vi "test Get-Set-Get Parameter Definitions.vi"(8 "error in":errorcluster, 11 "TestCase in":refnum<class "Scripting.lvclass">) -> (0 "error out":errorcluster, 3 "TestCase out":refnum<class "Scripting.lvclass">)   [LabVIEW 2023, in "Scripting.lvclass"]
uses:
  Scripting.lvclass
  <vilib>/addons/_JKI Toolkits/VI Tester/TestCase.llb/TestCase.lvclass
  Scripting/Ballard MIL-STD-1553 Scripting.lvlib
  Shared/Address.ctl
  Shared/Message Type.ctl
  Shared/Terminal Endpoint.ctl
  Shared/Parameter Definition.ctl
  Shared/Message Definition.ctl
  Shared/1553 Channel.ctl
  <vilib>/NI VeriStand/Custom Device API/Custom Device API.lvlib
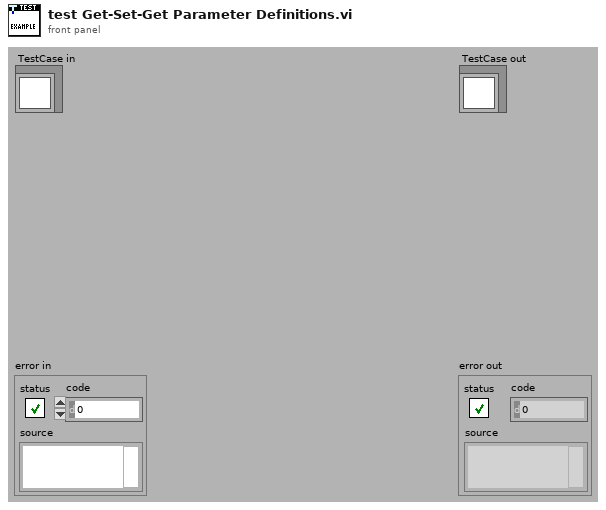
[diagram p1: front panel]
types:
  T1 = typedef "1553 Channel.ctl" = cluster{"HW channel":u16, "bus controller":cluster{"simulated?":bool, "name":string}, "terminal addresses":T2[], "terminal names":string[], "acyclic frame names":string[], "messages":T3[]}
  T2 = typedef "Address.ctl" = u16
  T3 = typedef "Message Definition.ctl" = cluster{"name":string, "message type":T4, "endpoint Tx":T5, "endpoint Rx":T5, "create timestamp channel":bool, "mode code":u16, "number of words":u16, "parameters":cluster{"name":string, "default value":dbl, "unit":string, "parameter definition":T6}[]}
  T4 = typedef "Message Type.ctl" = string
  T5 = typedef "Terminal Endpoint.ctl" = cluster{"terminal address":T2, "subaddress":T2}
  T6 = typedef "Parameter Definition.ctl" = cluster{"start index":i32, "size (bits)":i32, "encoding":enum16{"BNR", "BCD", "Discrete"}, "signed":bool, "multiplier":dbl, "offset":dbl}
  T7 = typedef "Custom Device API.lvlib/Custom Device Item Ref.ctl" = u64
  T8 = cluster{"name":string, "default value":dbl, "unit":string, "parameter definition":T6}[]
  T9 = typedef "Custom Device API.lvlib/Custom Device Channel.ctl" = cluster{"Type":T10, "Units":string, "Default Value":dbl, "Faultable":bool, "Scalable":bool}
  T10 = typedef "Custom Device API.lvlib/Custom Device Channel Type.ctl" = enum16{"Input", "Output"}
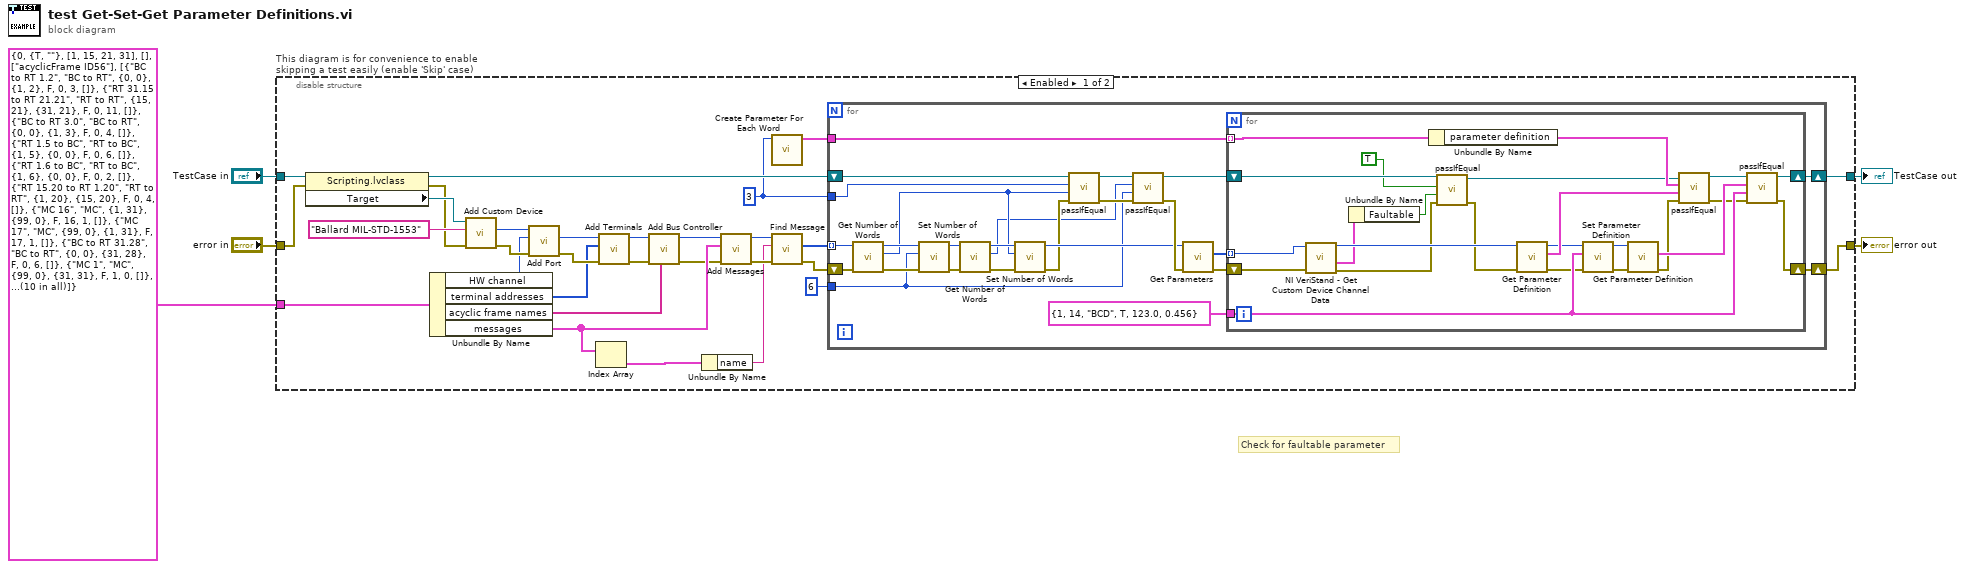
[diagram p0: block diagram]
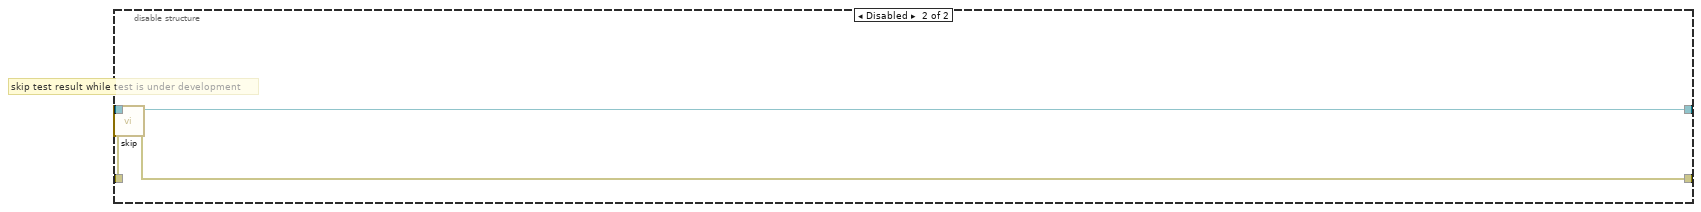
[diagram p2: hidden frame]
diagram:
  # "Check for faultable parameter"
  n1 = disable-structure "This diagram is for convenience to enable skipping a test easily (enable 'Skip' case)" shown="Enabled" {
    disable-tunnel: "TestCase in" -> [w34 w88]
    disable-tunnel: [w15 w86] -> w2
    disable-tunnel: [w14 w87] -> w4
    disable-tunnel: "error in" -> [w19 w85]
    disable-tunnel: T1 {"HW channel"=0, "bus controller"={"simulated?"=TRUE, "name"=""}, "terminal addresses"=[1, 15, 21, 31], "terminal names"=[], "acyclic frame names"=["acyclicFrame ID56"], "messages"=[{"name"="BC to RT 1.2", "message type"="BC to RT", "endpoint Tx"={"terminal address"=0, "subaddress"=0}, "endpoint Rx"={"terminal address"=1, "subaddress"=2}, "create timestamp channel"=FALSE, "mode code"=0, "number of words"=3, "parameters"=[]}, {"name"="RT 31.15 to RT 21.21", "message type"="RT to RT", "endpoint Tx"={"terminal address"=15, "subaddress"=21}, "endpoint Rx"={"terminal address"=31, "subaddress"=21}, "create timestamp channel"=FALSE, "mode code"=0, "number of words"=11, "parameters"=[]}, {"name"="BC to RT 3.0", "message type"="BC to RT", "endpoint Tx"={"terminal address"=0, "subaddress"=0}, "endpoint Rx"={"terminal address"=1, "subaddress"=3}, "create timestamp channel"=FALSE, "mode code"=0, "number of words"=4, "parameters"=[]}, {"name"="RT 1.5 to BC", "message type"="RT to BC", "endpoint Tx"={"terminal address"=1, "subaddress"=5}, "endpoint Rx"={"terminal address"=0, "subaddress"=0}, "create timestamp channel"=FALSE, "mode code"=0, "number of words"=6, "parameters"=[]}, {"name"="RT 1.6 to BC", "message type"="RT to BC", "endpoint Tx"={"terminal address"=1, "subaddress"=6}, "endpoint Rx"={"terminal address"=0, "subaddress"=0}, "create timestamp channel"=FALSE, "mode code"=0, "number of words"=2, "parameters"=[]}, {"name"="RT 15.20 to RT 1.20", "message type"="RT to RT", "endpoint Tx"={"terminal address"=1, "subaddress"=20}, "endpoint Rx"={"terminal address"=15, "subaddress"=20}, "create timestamp channel"=FALSE, "mode code"=0, "number of words"=4, "parameters"=[]}, {"name"="MC 16", "message type"="MC", "endpoint Tx"={"terminal address"=1, "subaddress"=31}, "endpoint Rx"={"terminal address"=99, "subaddress"=0}, "create timestamp channel"=FALSE, "mode code"=16, "number of words"=1, "parameters"=[]}, {"name"="MC 17", "message type"="MC", "endpoint Tx"={"terminal address"=99, "subaddress"=0}, "endpoint Rx"={"terminal address"=1, "subaddress"=31}, "create timestamp channel"=FALSE, "mode code"=17, "number of words"=1, "parameters"=[]}, {"name"="BC to RT 31.28", "message type"="BC to RT", "endpoint Tx"={"terminal address"=0, "subaddress"=0}, "endpoint Rx"={"terminal address"=31, "subaddress"=28}, "create timestamp channel"=FALSE, "mode code"=0, "number of words"=6, "parameters"=[]}, {"name"="MC 1", "message type"="MC", "endpoint Tx"={"terminal address"=99, "subaddress"=0}, "endpoint Rx"={"terminal address"=31, "subaddress"=31}, "create timestamp channel"=FALSE, "mode code"=1, "number of words"=0, "parameters"=[]}]} ("1553 channel") -> [w11 _]
    frame Enabled {
      w17 = u16 3 ("number of words")
      n2 = property class="Scripting.lvclass"(reference=w34, error in=w19) -> (reference out=w20:refnum<class "Scripting.lvclass">, error out=w18:errorcluster, "Target"=w33:refnum<k24>)
      n3 = Unbundle By Name(w11) -> ("HW channel"=w29:u16, "terminal addresses"=w26:T2[], "acyclic frame names"=w6:string[], "messages"=w12:T3[])
      n4 = call "Add Custom Device.vi"("error in"=w18, "name"="Ballard MIL-STD-1553", "target in"=w33) -> ("error out"=w32:errorcluster, "Ballard MIL-STD 1553 custom device"=w31:T7)  [unwired: 6 in, 1 out]
      n5 = call "Add Port.vi"("error in"=w32, "port number"=w29, "Ballard MIL-STD 1553 custom device in"=w31) -> ("error out"=w27:errorcluster, "port"=w28:T7)  [unwired: 6 in, 1 out]
      n6 = Index Array(array=w12) -> (element=w23:T3)  [unwired: 1 in]
      n7 = call "Add Terminals.vi"("error in"=w27, "terminal addresses"=w26, "port in"=w28) -> ("error out"=w10:errorcluster, "port out"=w9:T7)  [unwired: 7 in]
      n8 = call "Add Bus Controller.vi"("acyclic frame names"=w6, "error in"=w10, "port in"=w9) -> ("error out"=w7:errorcluster, "port out"=w8:T7)  [unwired: 6 in, 1 out]
      n9 = Unbundle By Name(w23) -> ("name"=w24:string)
      n10 = call "Add Messages.vi"("error in"=w7, "messages"=w12, "port in"=w8) -> ("error out"=w25:errorcluster, "port out"=w30:T7)  [unwired: 7 in]
      n11 = call "Create Parameter For Each Word.vi"("number of words"=w17) -> ("parameters"=w16:T8)  [unwired: 9 in, 1 out]
      n12 = call "Find Message.vi"("error in"=w25, "message name"=w24, "port in"=w30) -> ("error out"=w21:errorcluster, "message refs"=w22:T7[])  [unwired: 5 in, 2 out]
      n13 = for {
        tunnel: w22 -> [w60] mode=indexing
        shift-right: [w45] -> w14
        shift-left: w21 -> [w59]
        shift-right: [w46] -> w15
        shift-left: w20 -> [w52]
        tunnel: w17 -> [w40]
        tunnel: w16 -> [w48]
        tunnel: u16 6 ("number of words") -> [w37]
        n14 = call "Get Number of Words.vi"("error in"=w59, "message in"=w60) -> ("error out"=w57:errorcluster, "number of words"=w38:u16, "message out"=w58:T7)  [unwired: 7 in]
        n15 = call "Set Number of Words.vi"("error in"=w57, "number of words"=w37, "message in"=w58) -> ("error out"=w56:errorcluster, "message out"=w55:T7)  [unwired: 7 in]
        n16 = call "Get Number of Words.vi"("error in"=w56, "message in"=w55) -> ("error out"=w42:errorcluster, "number of words"=w36:u16, "message out"=w44:T7)  [unwired: 7 in]
        n17 = call "Set Number of Words.vi"("error in"=w42, "number of words"=w38, "message in"=w44) -> ("error out"=w41:errorcluster, "message out"=w43:T7)  [unwired: 7 in]
        n18 = call-dynamic "passIfEqual.vi"("error in (no error)"=w41, "y"=w38, "x"=w40, "TestCase in"=w52) -> ("error out"=w54:errorcluster, "TestCase out"=w53:refnum<class "Scripting.lvclass">)  [unwired: 6 in]
        n19 = call-dynamic "passIfEqual.vi"("error in (no error)"=w54, "y"=w37, "x"=w36, "TestCase in"=w53) -> ("error out"=w51:errorcluster, "TestCase out"=w47:refnum<class "Scripting.lvclass">)  [unwired: 6 in]
        n20 = call "Get Parameters.vi"("error in"=w51, "message in"=w43) -> ("error out"=w50:errorcluster, "parameters"=w49:T7[])  [unwired: 7 in, 1 out]
        n21 = for {
          shift-right: [w76] -> w45
          shift-left: w50 -> [w70]
          tunnel: w49 -> [w68] mode=indexing
          tunnel: w48 -> [w75] mode=indexing
          shift-right: [w77] -> w46
          shift-left: w47 -> [w66]
          tunnel: T6 {"start index"=1, "size (bits)"=14, "encoding"=enum."BCD", "signed"=TRUE, "multiplier"=123.0, "offset"=0.456} ("parameter definition") -> [w79]
          n22 = call <vilib>:"NI VeriStand - Get Custom Device Channel Data.vi"("error in (no error)"=w70, "Channel Ref in"=w68) -> ("error out"=w62:errorcluster, "Channel"=w67:T9, "Channel Ref out"=w69:T7)  [unwired: 4 in, 3 out]
          n23 = Unbundle By Name(w67) -> ("Faultable"=w64:bool)
          n24 = Unbundle By Name(w75) -> ("parameter definition"=w71:T6)
          n25 = call-dynamic "passIfEqual.vi"("error in (no error)"=w62, "y"=w64, "x"=TRUE ("Faultable"), "TestCase in"=w66) -> ("error out"=w61:errorcluster, "TestCase out"=w65:refnum<class "Scripting.lvclass">)  [unwired: 6 in]
          n26 = call "Get Parameter Definition.vi"("error in"=w61, "parameter in"=w69) -> ("error out"=w73:errorcluster, "parameter definition"=w84:T6, "parameter out"=w83:T7)  [unwired: 7 in]
          n27 = call "Set Parameter Definition.vi"("error in"=w73, "parameter definition"=w79, "parameter in"=w83) -> ("error out"=w81:errorcluster, "parameter out"=w82:T7)  [unwired: 7 in]
          n28 = call "Get Parameter Definition.vi"("error in"=w81, "parameter in"=w82) -> ("error out"=w72:errorcluster, "parameter definition"=w80:T6)  [unwired: 7 in, 1 out]
          n29 = call-dynamic "passIfEqual.vi"("error in (no error)"=w72, "y"=w84, "x"=w71, "TestCase in"=w65) -> ("error out"=w74:errorcluster, "TestCase out"=w78:refnum<class "Scripting.lvclass">)  [unwired: 6 in]
          n30 = call-dynamic "passIfEqual.vi"("error in (no error)"=w74, "y"=w79, "x"=w80, "TestCase in"=w78) -> ("error out"=w76:errorcluster, "TestCase out"=w77:refnum<class "Scripting.lvclass">)  [unwired: 6 in]
        }
      }
    }
    frame Disabled {
      # "skip test result while test is under development"
      n31 = call <vilib>:"skip.vi"("error in (no error)"=w85, "TestCase in"=w88) -> ("error out"=w87:errorcluster, "TestCase out"=w86:refnum<class "Scripting.lvclass">)  [unwired: 8 in]
    }
  }
  "error out" <- w4
  "TestCase out" <- w2
